vi "Open VI by path.vi"(8 "error in (no error)":errorcluster, 10 "vi path":path, 11 "LV RT in":refnum<class "LV RT.lvclass">) -> (0 "error out":errorcluster, 3 "LV RT out":refnum<class "LV RT.lvclass">)   [LabVIEW 2016, in "LV RT.lvclass"]
uses:
  LV RT.lvclass
  D:/Navin Workspace/MDI/source code/Document/LV Doc/LV Doc.lvclass
  LV Doc.lvclass/LV Doc.ctl
  LV RT.lvclass/LV RT.ctl
  property/Write VI Reference.vi
  property/Write Instantiated by ref_.vi
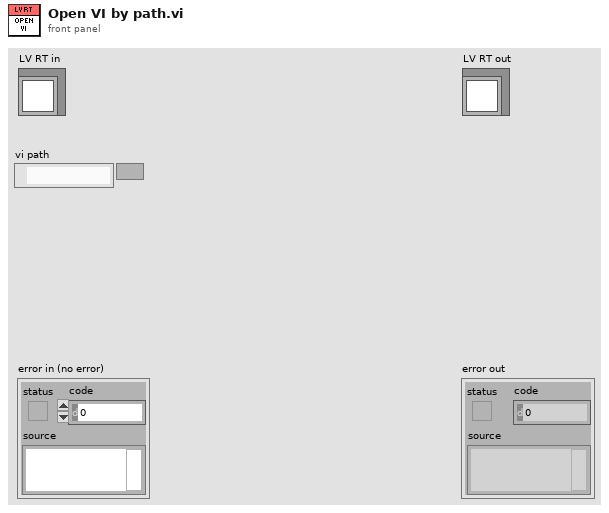
[diagram p1: front panel]
types:
  T1 = enum32{"Invalid", "Standard", "Closed", "Hidden", "Minimized", "Maximized"}
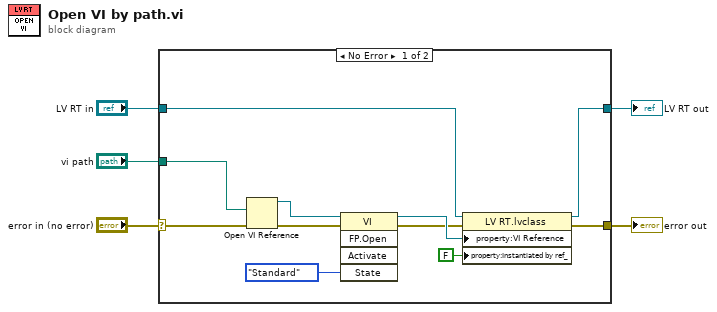
[diagram p0: block diagram]
diagram:
  n1 = case shown="No Error" "error in (no error)" {
    selector: "error in (no error)" -> [w7 w18]
    tunnel: [w8 w18] -> w4
    tunnel: [w10 w17] -> w2
    tunnel: "LV RT in" -> [w11 w17]
    tunnel: "vi path" -> [w13 _]
    frame No Error {
      n2 = Open VI Reference(vi path=w13, error in (no error)=w7) -> (vi reference=w15:refnum<vi>, error out=w14:errorcluster)  [unwired: 4 in]
      n3 = invoke class="VI" method="FP.Open"(reference=w15, error in=w14, "State"=T1."Standard") -> (reference out=w12:refnum<vi>, error out=w9:errorcluster)  [unwired: 2 in, 3 out]
      n4 = property class="LV RT.lvclass"(reference=w11, error in=w9, "property:VI Reference"=w12, "property:Instantiated by ref_"=FALSE ("Instantiated by ref_")) -> (reference out=w10:refnum<class "LV RT.lvclass">, error out=w8:errorcluster)
    }
    frame Error {
    }
  }
  "error out" <- w4
  "LV RT out" <- w2
